vi "DestroySelfReference.vi"(8 "error in (no error)":errorcluster, 11 "DAQ_UI":refnum<class "DAQ_UI.lvclass">) -> (0 "error out":errorcluster, 3 "DAQ_UI out":refnum<class "DAQ_UI.lvclass">)   [LabVIEW 2020, in "DAQ_UI.lvclass"]
doc: "JKI State Machine Objects (SMO) 1.0.0.5\nJKI - JKI\nCopyright (c) 2016, JKI"
uses:
  DAQ_UI.lvclass
  DAQ_UI.lvclass/DAQ_UI.ctl
  <vilib>/JKI/JKI SMO/SMO.UI/SMO.UI.lvclass
panel:
  # "For instructions on how to use the JKI State Machine Objects, examples and video tutorials, visit:\nhttp://jki.net/state-machine-objects/\n\nJKI State Machine Objects™\nhttp://jki.net/state-machine-objects/\nCopyright (C) 2005-2015, JKI <info@jki.net>\nALL RIGHTS RESERVED"
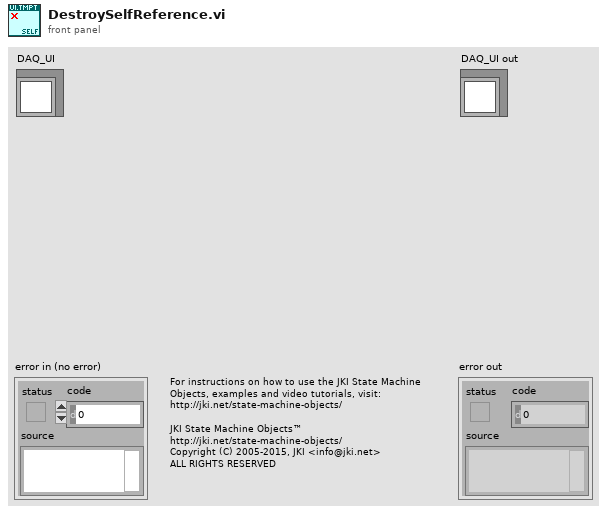
[diagram p1: front panel]
types:
  T1 = typedef "DAQ_UI.lvclass/PrivateData--Ref.ctl" = refnum<data-value>
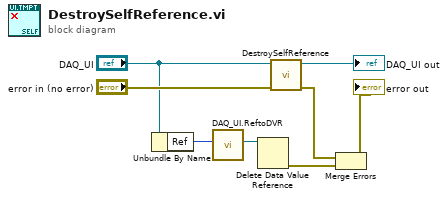
[diagram p0: block diagram]
diagram:
  n1 = Unbundle By Name("DAQ_UI") -> ("Ref"=w2:u32)
  n2 = call "DAQ_UI.ReftoDVR.vi"("Ref"=w2) -> ("Ref"=w1:T1)  [unwired: 10 in]
  n3 = Delete Data Value Reference(data value reference=w1) -> (error out=w5:errorcluster)  [unwired: 1 in, 1 out]
  n4 = call-parent "DestroySelfReference.vi"("error in (no error)"="error in (no error)", "SMO.UI"="DAQ_UI") -> ("error out"=w4:errorcluster, "SMO.UI out"=→"DAQ_UI out":refnum<class "DAQ_UI.lvclass">)  [unwired: 8 in]
  n5 = Merge Errors(w4, w5) -> (→"error out":errorcluster)
